vi "Get MSS.vi"(11 "Series Base in":refnum<class "Series Base.lvclass">) -> (2 "Measure and Stimulus Subsystems":refnum<class "Measure and Stimulus Subsystems.lvclass">, 3 "Series Base out":refnum<class "Series Base.lvclass">)   [LabVIEW 2023, in "Series Base.lvclass"]
uses:
  Series Base.lvclass
  Measure and Stimulus Subsystems/Measure and Stimulus Subsystems.lvclass
  Series Base.lvclass/Series Base.ctl
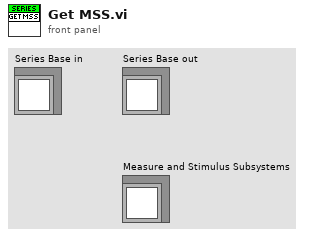
[diagram p1: front panel]
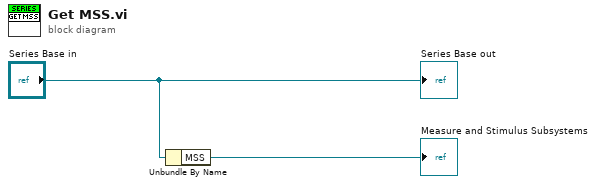
[diagram p0: block diagram]
diagram:
  n1 = Unbundle By Name("Series Base in") -> ("MSS"=→"Measure and Stimulus Subsystems":refnum<class "Measure and Stimulus Subsystems.lvclass">)
  "Series Base out" <- "Series Base in"
